vi "Macro Builder.vi"(9 "Module Code (do not add sub and end sub)":string, 10 "Module Name":string, 11 "Type":enum16{"FUNCTION", "SUB"}(ring)) -> (1 "concatenated string":string)   [LabVIEW 2016]
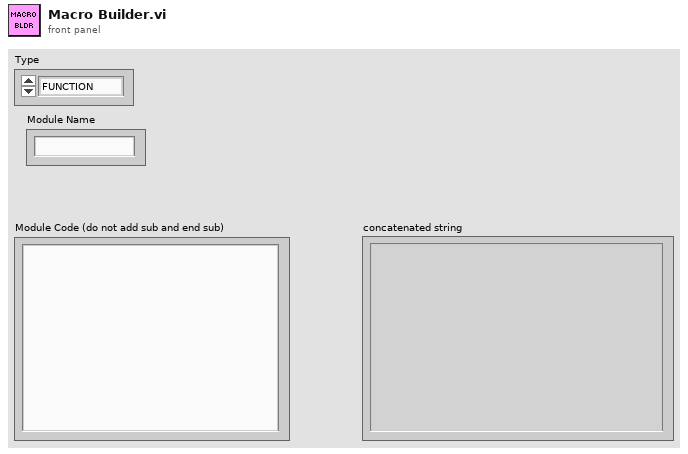
[diagram p1: front panel]
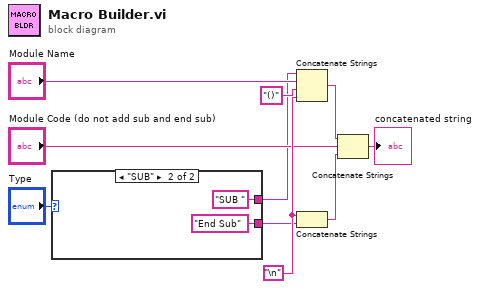
[diagram p0: block diagram]
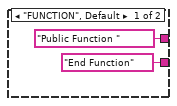
[diagram p2: hidden frame]
diagram:
  w8 = "\n"
  n1 = case shown="\"SUB\"" "Type" {
    tunnel: ["Public Function " ("string") "SUB " ("string")] -> w2
    tunnel: ["End Function" ("string") "End Sub" ("string")] -> w1
    frame "FUNCTION", Default {
    }
    frame "SUB" {
    }
  }
  n2 = Concatenate Strings(w2, "Module Name", "()" ("string"), w8) -> (w9:string)
  n3 = Concatenate Strings(w8, w1) -> (w7:string)
  n4 = Concatenate Strings(w9, "Module Code (do not add sub and end sub)", w7) -> (→"concatenated string":string)
